vi "DAQ AI Configuration Settting.vi"(8 "DO Channel Setting":T1, 9 "DI Channel Setting":T2, 10 "AO Channel Setting":T3={"AO Channel name"=[], "output terminal configuration"=enum."RSE", "minimum value"=-10.0, "maximum value"=10.0, "units"=enum."Volts", "name to assign"=[]} {"maximum value" format="%0.2f"; "minimum value" format="%0.2f"}, 11 "AI Setting":T4={"Physical Channel"=["6363/ai0", "6363/ai1", "6363/ai2", "6363/ai2"], "Name to assign"=["AI_1", "AI_2", "AI_3", "AI_4"], "input terminal configuration"=enum."RSE", "minimum value"=0.0, "maximum value"=10.0, "units"=enum."Volts", "custom scale name"="Motor_speed", "sample mode"=enum."Finite Samples", "rate"=5000.0, "samples per channel"=1000.0} {"rate" format="%#_13g"; "maximum value" format="%#_13g"; "minimum value" format="%#_13g"}) -> (0 "DAQ DO Parameter":string, 1 "DAQ DI Parameter":string, 2 "DAQ AO Parameter":string[](array[string]), 3 "DAQ AI Parameter":string[](array[string]))   [LabVIEW 2016, in "User Interface.lvlib"]
uses:
  User Interface.lvlib
  AI Channel Setting.ctl
  DAQ Hardware/DAQ Hardware.lvlib
  DAQ Hardware/AO Channel Setting.ctl
  DAQ Hardware/DI Channel Setting.ctl
  DAQ Hardware/DO Channel Setting.ctl
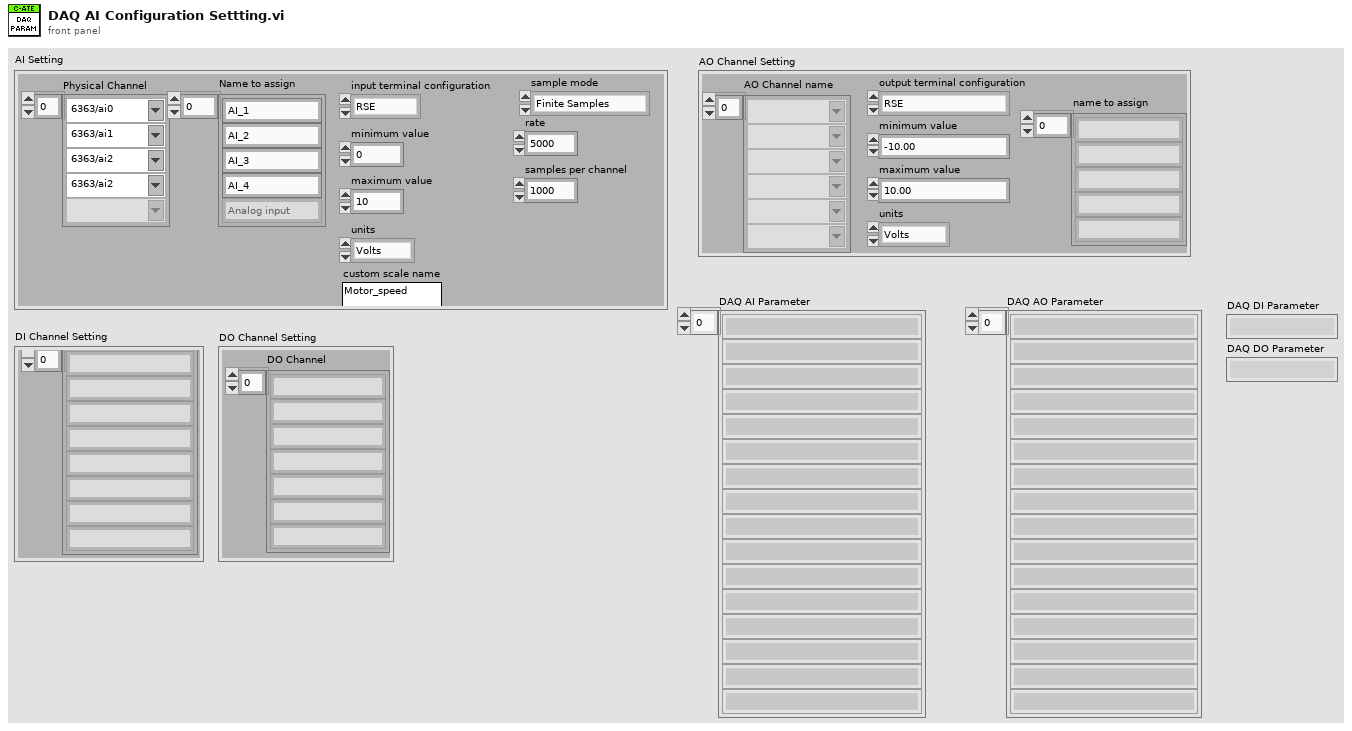
[diagram p1: front panel]
types:
  T1 = typedef "DAQ Hardware.lvlib/DO Channel Setting.ctl" = cluster{"DO Channel":string[]}
  T2 = typedef "DAQ Hardware.lvlib/DI Channel Setting.ctl" = cluster{"DI Channel":string[]}
  T3 = typedef "DAQ Hardware.lvlib/AO Channel Setting.ctl" = cluster{"AO Channel name":string[], "output terminal configuration":enum16{"RSE", "NRSE", "Differential"}, "minimum value":dbl, "maximum value":dbl, "units":enum16{"Volts"}, "name to assign":string[]}
  T4 = typedef "DAQ Hardware.lvlib/AI Channel Setting.ctl" = cluster{"Physical Channel":string[], "Name to assign":string[], "input terminal configuration":enum16{"RSE", "NRSE", "Differential"}, "minimum value":dbl, "maximum value":dbl, "units":enum16{"Volts"}, "custom scale name":string, "sample mode":enum16{"Finite Samples", "Continuous Samples", "Hardware Timed Single Point"}, "rate":dbl, "samples per channel":dbl}
  T5 = enum16{"Finite Samples", "Continuous Samples", "Hardware Timed Single Point"}
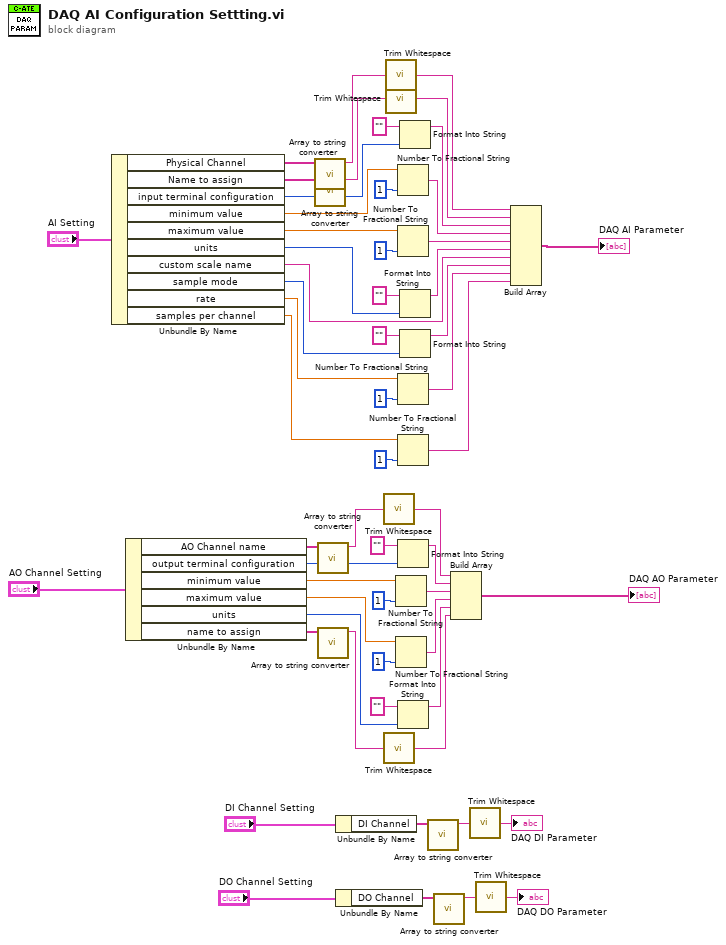
[diagram p0: block diagram]
diagram:
  n1 = Unbundle By Name("AI Setting") -> ("Physical Channel"=w43:string[], "Name to assign"=w41:string[], "input terminal configuration"=w15:enum16{"RSE", "NRSE", "Differential"}, "minimum value"=w57:dbl, "maximum value"=w55:dbl, "units"=w11:enum16{"Volts"}, "custom scale name"=w47:string, "sample mode"=w8:T5, "rate"=w52:dbl, "samples per channel"=w50:dbl)
  n2 = Unbundle By Name("AO Channel Setting") -> ("AO Channel name"=w36:string[], "output terminal configuration"=w5:enum16{"RSE", "NRSE", "Differential"}, "minimum value"=w32:dbl, "maximum value"=w31:dbl, "units"=w2:enum16{"Volts"}, "name to assign"=w26:string[])
  n3 = call "Array to string converter.vi"("Data In"=w43) -> ("Data Out"=w42:string)  [unwired: 10 in]
  n4 = call "Array to string converter.vi"("Data In"=w41) -> ("Data Out"=w40:string)  [unwired: 10 in]
  n5 = call "Array to string converter.vi"("Data In"=w36) -> ("Data Out"=w35:string)  [unwired: 10 in]
  n6 = call "Array to string converter.vi"("Data In"=w26) -> ("Data Out"=w27:string)  [unwired: 10 in]
  n7 = Unbundle By Name("DI Channel Setting") -> ("DI Channel"=w21:string[])
  n8 = Unbundle By Name("DO Channel Setting") -> ("DO Channel"=w17:string[])
  n9 = call <vilib>:"Trim Whitespace.vi"("string"=w35) -> ("trimmed string"=w30:string)  [unwired: 1 in]
  n10 = call <vilib>:"Trim Whitespace.vi"("string"=w27) -> ("trimmed string"=w25:string)  [unwired: 1 in]
  n11 = call <vilib>:"Trim Whitespace.vi"("string"=w42) -> ("trimmed string"=w39:string)  [unwired: 1 in]
  n12 = call <vilib>:"Trim Whitespace.vi"("string"=w40) -> ("trimmed string"=w38:string)  [unwired: 1 in]
  n13 = Number To Fractional String(number=w32, precision (6)=i16 1) -> (F-format string=w29:string)  [unwired: 2 in]
  n14 = Number To Fractional String(number=w31, precision (6)=i16 1) -> (F-format string=w28:string)  [unwired: 2 in]
  n15 = Number To Fractional String(number=w57, precision (6)=i16 1) -> (F-format string=w49:string)  [unwired: 2 in]
  n16 = Number To Fractional String(number=w55, precision (6)=i16 1) -> (F-format string=w48:string)  [unwired: 2 in]
  n17 = Number To Fractional String(number=w52, precision (6)=i16 1) -> (F-format string=w46:string)  [unwired: 2 in]
  n18 = Number To Fractional String(number=w50, precision (6)=i16 1) -> (F-format string=w45:string)  [unwired: 2 in]
  n19 = Format Into String(initial string="", w5) -> (resulting string=w4:string)  [unwired: 2 in, 1 out]
  n20 = Format Into String(initial string="", w2) -> (resulting string=w1:string)  [unwired: 2 in, 1 out]
  n21 = Format Into String(initial string="", w15) -> (resulting string=w13:string)  [unwired: 2 in, 1 out]
  n22 = Format Into String(initial string="", w11) -> (resulting string=w10:string)  [unwired: 2 in, 1 out]
  n23 = Format Into String(initial string="", w8) -> (resulting string=w7:string)  [unwired: 2 in, 1 out]
  n24 = call "Array to string converter.vi"("Data In"=w21) -> ("Data Out"=w22:string)  [unwired: 10 in]
  n25 = call "Array to string converter.vi"("Data In"=w17) -> ("Data Out"=w18:string)  [unwired: 10 in]
  n26 = Build Array(w30, w4, w29, w28, w1, w25) -> (→"DAQ AO Parameter":string[])
  n27 = call <vilib>:"Trim Whitespace.vi"("string"=w22) -> ("trimmed string"=→"DAQ DI Parameter":string)  [unwired: 1 in]
  n28 = call <vilib>:"Trim Whitespace.vi"("string"=w18) -> ("trimmed string"=→"DAQ DO Parameter":string)  [unwired: 1 in]
  n29 = Build Array(w39, w38, w13, w49, w48, w10, w47, w7, w46, w45) -> (→"DAQ AI Parameter":string[])
